vi "Load System.vi"(8 "Buttons 2":T1, 9 "Buttons":T1, 10 "Axes":T2) -> ()   [LabVIEW 2012]
uses:
  <vilib>/Rock Robotics/WPI/Joystick/WPI_JoystickButtonState.ctl
  <vilib>/Rock Robotics/WPI/Solenoid/Deprecated/WPI_SolenoidSetBool.vi
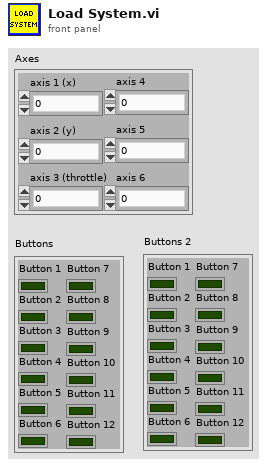
[diagram p1: front panel]
types:
  T1 = typedef "WPI_JoystickButtonState.ctl" = cluster{"Button 1":bool, "Button 2":bool, "Button 3":bool, "Button 4":bool, "Button 5":bool, "Button 6":bool, "Button 7":bool, "Button 8":bool, "Button 9":bool, "Button 10":bool, "Button 11":bool, "Button 12":bool}
  T2 = cluster{"axis 1 (x)":dbl, "axis 2 (y)":dbl, "axis 3 (throttle)":dbl, "axis 4":dbl, "axis 5":dbl, "axis 6":dbl}
  T3 = typedef "WPI_MotorControlDeviceRef.ctl" = cluster{"DeviceStatus":errorcluster, "Type":enum16{"PWM", "CAN"}, "PWM":cluster{"Digital Module":T4, "PWM Channel":T5, "DeadBand":T6}, "CAN":cluster{"Device Number":u8, "Control Mode":T7, "Semaphore":T8, "Max Vout":dbl}, "Invert":bool, "TransformRef":T9, "InvTransformRef":T9}
  T4 = typedef "FPGA_TypedefDigitalModule.ctl" = enum16{"Digital Module 1", "Digital Module 2"}
  T5 = typedef "FPGA_DIOPWMChannel.ctl" = enum8{"PWM 1", "PWM 2", "PWM 3", "PWM 4", "PWM 5", "PWM 6", "PWM 7", "PWM 8", "PWM 9", "PWM 10", "Invalid"}
  T6 = typedef "WPI_PWMDeadband.ctl" = cluster{"Name":string, "maxPositivePwm":i32, "minPositivePwm":i32, "centerPwm":i32, "maxNegativePwm":i32, "minNegativePwm":i32, "angularRange":u16}
  T7 = typedef "WPI_CANJaguar_ControlMode.ctl" = enum8{"Percent VBus", "Current", "Speed", "Position", "Voltage"}
  T8 = typedef "Semaphore RefNum" = refnum<k1>
  T9 = typedef "WPI_PWMTransform_ConPane.ctl" = refnum<vi>
  T10 = typedef "WPI_SolenoidDevRef.ctl" = cluster{"DevStatus":errorcluster, "Solenoid Module":T11, "Forward Solenoid Channel":T12, "Reverse Solenoid Channel":T12}
  T11 = typedef "FPGA_TypedefSolenoidModule.ctl" = enum16{"Solenoid Module 1", "Solenoid Module 2"}
  T12 = typedef "WPI_SolenoidChannel.ctl" = enum8{"Solenoid 1", "Solenoid 2", "Solenoid 3", "Solenoid 4", "Solenoid 5", "Solenoid 6", "Solenoid 7", "Solenoid 8", "Invalid"}
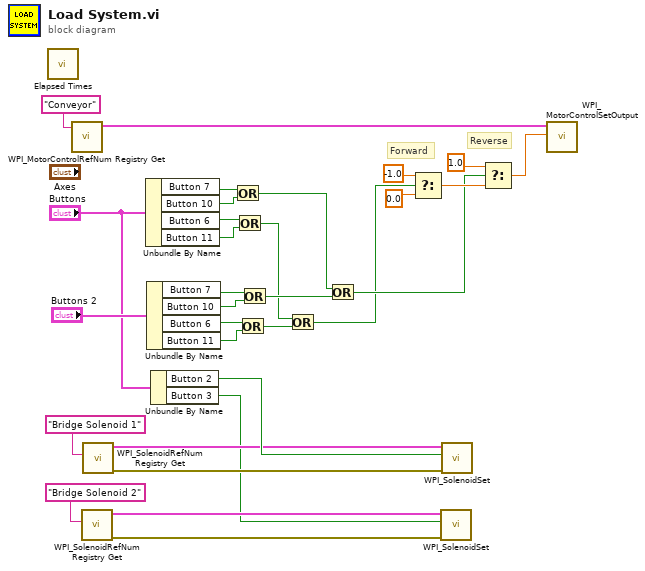
[diagram p0: block diagram]
diagram:
  # "Reverse"
  # "Forward"
  n1 = call "Elapsed Times.vi"() -> ()  [unwired: 3 in, 1 out]
  n2 = call <vilib>:"WPI_MotorControlRefNum Registry Get.vi"("refnum name"="Conveyor") -> ("MotorControlDevRef"=w29:T3)  [unwired: 9 in, 1 out]
  n3 = call <vilib>:"WPI_SolenoidRefNum Registry Get.vi"("refnum name"="Bridge Solenoid 2") -> ("error out"=w2:errorcluster, "SolenoidDevRef"=w3:T10)  [unwired: 9 in]
  n4 = call <vilib>:"WPI_SolenoidRefNum Registry Get.vi"("refnum name"="Bridge Solenoid 1") -> ("error out"=w7:errorcluster, "SolenoidDevRef"=w5:T10)  [unwired: 9 in]
  n5 = Unbundle By Name("Buttons") -> ("Button 7"=w24:bool, "Button 10"=w23:bool, "Button 6"=w22:bool, "Button 11"=w21:bool)
  n6 = Unbundle By Name("Buttons 2") -> ("Button 7"=w19:bool, "Button 10"=w18:bool, "Button 6"=w17:bool, "Button 11"=w16:bool)
  n7 = Unbundle By Name("Buttons") -> ("Button 2"=w6:bool, "Button 3"=w1:bool)
  n8 = Or(x=w24, y=w23) -> (x .or. y?=w15:bool)
  n9 = Or(x=w22, y=w21) -> (x .or. y?=w12:bool)
  n10 = Or(x=w17, y=w16) -> (x .or. y?=w11:bool)
  n11 = Or(x=w19, y=w18) -> (x .or. y?=w14:bool)
  n12 = Or(x=w12, y=w11) -> (x .or. y?=w10:bool)
  n13 = Or(x=w15, y=w14) -> (x .or. y?=w13:bool)
  n14 = Select(t=-1.0, s=w10, f=0.0) -> (s? t:f=w26:dbl)
  n15 = call-poly <vilib>:"WPI_SolenoidSet.vi"("error in (no error)"=w2, "Value"=w1, "SolenoidDevRef"=w3) -> ()  [unwired: 7 in, 2 out]
  n16 = call-poly <vilib>:"WPI_SolenoidSet.vi"("error in (no error)"=w7, "Value"=w6, "SolenoidDevRef"=w5) -> ()  [unwired: 7 in, 2 out]
  n17 = Select(t=1.0, s=w13, f=w26) -> (s? t:f=w25:dbl)
  n18 = call <vilib>:"WPI_MotorControlSetOutput.vi"("Output"=w25, "MotorControlDevRef"=w29) -> ()  [unwired: 7 in, 3 out]
